vi "HFRR ADV v02.vi"() -> ()   [LabVIEW 2025] (continued)
            n899 = local write "Temperature Selection"(T15."Default" ("Temperature Selection")) -> ()
            n900 = local write "Calibration Selection"(T10."Default" ("Calibration Selection")) -> ()
            n901 = local write "Friction Force Tab"(T13."Page 1" ("Friction Force Tab")) -> ()
            n902 = local write "Main Calibration Tab"(T9."Main" ("Main Calibration Tab")) -> ()
            n903 = property on="Tab Control 6" class="TabCtl (strict)"("Visible"=FALSE) -> ()  [unwired: 2 in, 2 out]
            n904 = property on="Friction Force Calibration Result Tab" class="TabCtl (strict)"("Visible"=FALSE) -> ()  [unwired: 2 in, 2 out]
          }
        }
      }
      event "Accept & Save FF": Value Change {
        n905 = event-data() -> ()  [unwired: 1 in, 6 out]
        n906 = stacked-sequence {
          frame #0 {
            n907 = Wait (ms)(milliseconds to wait=u32 1000) -> ()  [unwired: 1 out]
          }
          frame #1 {
            n908 = local write "Due Write"("VC;0") -> ()
          }
          frame #2 {
            n909 = Wait (ms)(milliseconds to wait=u32 1000) -> ()  [unwired: 1 out]
          }
          frame #3 {
            n910 = local write "Due Write"("VC;0") -> ()
          }
          frame #4 {
            w931 = FALSE
            n911 = local write "FF BACK 2"(w931) -> ()
            n912 = local write "FF BACK 3"(w931) -> ()
            n913 = local write "FF BACK 4"(w931) -> ()
            n914 = local write "FF BACK 5"(w931) -> ()
            n915 = local write "FF BACK 6"(w931) -> ()
            n916 = local write "FF BACK"(w931) -> ()
          }
          frame #5 {
            n917 = Get Date/Time In Seconds() -> (seconds since 1Jan1904=w934:timestamp)
            n918 = Format Into String(format string="%<%m/%d/%Y %I:%M:%S %p>T", w934) -> (resulting string=w932:string)  [unwired: 2 in, 1 out]
            n919 = local write "FRICTION CALIBRATION"(w932) -> ()
          }
          frame #6 {
            n920 = local write "Temperature Selection"(T15."Default" ("Temperature Selection")) -> ()
            n921 = local write "Calibration Selection"(T10."Default" ("Calibration Selection")) -> ()
            n922 = local write "Friction Force Tab"(T13."Page 1" ("Friction Force Tab")) -> ()
            n923 = local write "Main Calibration Tab"(T9."Main" ("Main Calibration Tab")) -> ()
            n924 = local write "Save Button"(TRUE ("Save Button")) -> ()
            n925 = property on="Tab Control 6" class="TabCtl (strict)"("Visible"=FALSE) -> ()  [unwired: 2 in, 2 out]
            n926 = property on="Friction Force Calibration Result Tab" class="TabCtl (strict)"("Visible"=FALSE) -> ()  [unwired: 2 in, 2 out]
          }
        }
      }
      event "FF CONTINUE": Value Change {
        n927 = event-data() -> ()  [unwired: 1 in, 6 out]
        n928 = local write "FF CONTINUE"(FALSE ("FF CONTINUE")) -> ()
        n929 = local write "Friction Force Tab"(T13."Page 2" ("Friction Force Tab")) -> ()
      }
      event "FF CONTINUE 2": Value Change {
        n930 = event-data() -> ()  [unwired: 1 in, 6 out]
        n931 = local write "FF CONTINUE 2"(FALSE ("FF CONTINUE")) -> ()
        n932 = local write "Friction Force Tab"(T13."Page 3" ("Friction Force Tab")) -> ()
      }
      event "FF CONTINUE 3": Value Change {
        n933 = event-data() -> ()  [unwired: 1 in, 6 out]
        n934 = local write "FF CONTINUE 3"(FALSE ("FF CONTINUE")) -> ()
        n935 = local write "Friction Force Tab"(T13."Page 4" ("Friction Force Tab")) -> ()
      }
      event "FF CONTINUE 4": Value Change {
        n936 = event-data() -> ()  [unwired: 1 in, 6 out]
        n937 = local write "FF CONTINUE 4"(FALSE ("FF CONTINUE")) -> ()
        n938 = local write "Friction Force Tab"(T13."Page 5" ("Friction Force Tab")) -> ()
        n939 = property on="Friction Force Calibration Result Tab" class="TabCtl (strict)"("Visible"=FALSE) -> ()  [unwired: 2 in, 2 out]
      }
      event "FF CONTINUE 5": Value Change {
        n940 = event-data() -> ()  [unwired: 1 in, 6 out]
        n941 = local write "FF CONTINUE 5"(FALSE ("FF CONTINUE")) -> ()
        n942 = local write "Friction Force Tab"(T13."Page 6" ("Friction Force Tab")) -> ()
        n943 = property on="Friction Force Calibration Result Tab" class="TabCtl (strict)"("Visible"=FALSE) -> ()  [unwired: 2 in, 2 out]
        n944 = property on="Tab Control 6" class="TabCtl (strict)"("Visible"=FALSE) -> ()  [unwired: 2 in, 2 out]
      }
      event "Stroke Report Button": Value Change {
        n945 = event-data() -> ()  [unwired: 1 in, 6 out]
        n946 = local read "Point 5 - 1.0 mm"() -> (w956:bool)
        n947 = case shown="False" w956 {
          tunnel: [0.8 1.0] -> w955
          frame False {
          }
          frame True {
          }
        }
        n948 = local read "Machine Serial Number"() -> (w959:string)
        n949 = local read "USERNAME"() -> (w957:string)
        n950 = local write "Stroke Report Button"(FALSE ("Stroke Report Button")) -> ()
        n951 = call "Stroke Calibration Report.vi"("measured_value"=w955, "operator_name"=w957, "Instrument_serial Number"=w959) -> ()  [unwired: 7 in, 2 out]
      }
      event "Sample Report Button": Value Change {
        n952 = event-data() -> ()  [unwired: 1 in, 6 out]
        n953 = local read "Machine Serial Number"() -> (w965:string)
        n954 = local read "Sample 0deg temp"() -> (w962:dbl)
        n955 = local read "Sample 60deg temp"() -> (w963:dbl)
        n956 = local read "USERNAME"() -> (w964:string)
        n957 = call "Temperature Calibration Report.vi"("measured_60"=w963, "measured_zero"=w962, "operator_name"=w964, "Instrument_serial Number"=w965) -> ()  [unwired: 6 in, 2 out]
        n958 = local write "Sample Report Button"(FALSE ("Sample Report Button")) -> ()
      }
      event "Report Button FF": Value Change {
        n959 = event-data() -> ()  [unwired: 1 in, 6 out]
        n960 = local read "FF PASS"() -> (w970:bool)
        n961 = local read "Machine Serial Number"() -> (w973:string)
        n962 = Select(t="PASS", s=w970, f="FAIL") -> (s? t:f=w967:string)
        n963 = local read "USERNAME"() -> (w972:string)
        n964 = call "FF Calibration Report.vi"("pass_or_fail"=w967, "operator_name"=w972, "Instrument_serial Number"=w973) -> ()  [unwired: 7 in, 2 out]
        n965 = local write "Report Button FF"(FALSE ("Sample Report Button")) -> ()
      }
      event "Air Temperature Report Button": Value Change {
        n966 = event-data() -> ()  [unwired: 1 in, 6 out]
        n967 = local read "Machine Serial Number"() -> (w978:string)
        n968 = local read "Air 0deg temp"() -> (w975:dbl)
        n969 = local read "Air 60deg temp"() -> (w976:dbl)
        n970 = local read "USERNAME"() -> (w977:string)
        n971 = call "Air Temperature Calibration Report.vi"("measured_60"=w976, "measured_zero"=w975, "operator_name"=w977, "Instrument_serial Number"=w978) -> ()  [unwired: 6 in, 2 out]
        n972 = local write "Air Temperature Report Button"(FALSE ("Sample Report Button")) -> ()
      }
      event "Quit": Value Change {
        n973 = event-data() -> ()  [unwired: 1 in, 6 out]
      }
    }
    n974 = Wait (ms)(milliseconds to wait=u32 100) -> ()  [unwired: 1 out]
  }
  n975 = while {
    shift-right: [w981] -> _
    shift-left: "Enum - Selector" -> [w982]
    stop <- w983 stop-if-true
    # "Auto Start Logic Loop"
    n976 = case shown="\"close\"" w982 {
      tunnel: [w986 w992 w1020 w1055 w1085 Auto_Start_enum."Exit" ("Enum - Selector") Auto_Start_enum."Init" ("Enum - Selector")] -> w981
      frame "Init", Default {
        n977 = local read "Auto Start Test"() -> (w985:bool)
        n978 = Select(t=Auto_Start_enum."Humidity & Temperature On" ("Enum - Selector"), s=w985, f=Auto_Start_enum."Init") -> (s? t:f=w986:T17)
      }
      frame "Humidity & Temperature On" {
        n979 = stacked-sequence {
          tunnel: [_ _ _ _ _ _ Auto_Start_enum."Reach point" ("Enum - Selector")] -> w989
          frame #0 {
            w994 = T19."Disabled and Grayed Out" ("Disabled")
            w995 = TRUE ("Heater Button")
            n980 = property on="Humidity" class="Bool (strict)"("DisabledEnum"=w994) -> ()  [unwired: 2 in, 2 out]
            n981 = property on="Heater Button" class="Bool (strict)"("DisabledEnum"=w994) -> ()  [unwired: 2 in, 2 out]
            n982 = local write "Heater Button"(w995) -> ()
            n983 = local write "Humidity"(w995) -> ()
            n984 = property on="Heater Button" class="Bool (strict)"("Val(Sgnl)"=TRUE ("Value (Signaling)")) -> ()  [unwired: 2 in, 2 out]
          }
          frame #1 {
            n985 = Wait (ms)(milliseconds to wait=u32 3000) -> ()  [unwired: 1 out]
          }
          frame #2 {
            n986 = local read "Set Temp"() -> (w1001:dbl)
            n987 = Number To Fractional String(number=w1001, precision (6)=i16 2) -> (F-format string=w998:string)  [unwired: 2 in]
            n988 = Concatenate Strings("ST;" ("Command"), w998) -> (w999:string)
            n989 = local write "Due Write"(w999) -> ()
          }
          frame #3 {
            n990 = Wait (ms)(milliseconds to wait=u32 1500) -> ()  [unwired: 1 out]
          }
          frame #4 {
            (unwired) i16 2 ("precision (6)")
            n991 = local read "WriteHumidity"() -> (w1003:string[])
            n992 = local read "Set Rh"() -> (w1006:dbl)
            n993 = Number To Fractional String(number=w1006) -> (F-format string=w1007:string)  [unwired: 3 in]
            n994 = Concatenate Strings("M;" ("new element/subarray"), w1007) -> (w1008:string)
            n995 = Insert Into Array(array=w1003, new element=w1008) -> (w1004:string[])  [unwired: 1 in]
            n996 = local write "WriteHumidity"(w1004) -> ()
            n997 = local write "Due Write"("HE;1" ("Command")) -> ()
          }
          frame #5 {
            n998 = Wait (ms)(milliseconds to wait=u32 1500) -> ()  [unwired: 1 out]
          }
          frame #6 {
            w1011 = TRUE ("Reach point temp")
            n999 = local write "Reach point Humidity"(w1011) -> ()
            n1000 = local write "Reach point temp"(w1011) -> ()
          }
        }
        n1001 = local read "Auto Start Test"() -> (w991:bool)
        n1002 = Not(x=w991) -> (.not. x?=w990:bool)
        n1003 = Select(t=Auto_Start_enum."close", s=w990, f=w989) -> (s? t:f=w992:T17)
      }
      frame "Reach point" {
        w1021 = TRUE ("PAUSE")
        w1029 = 1.0 ("y")
        w1032 = 1.0 ("y")
        n1004 = local read "Set Temp"() -> (w1014:dbl)
        n1005 = local read "Set Humidity:"() -> (w1028:dbl)
        n1006 = local read "Humidity ( %RH )"() -> (w1033:dbl)
        n1007 = Add(x=w1014, y=w1032) -> (x+y=w1031:dbl)
        n1008 = Subtract(x=w1014, y=w1032) -> (x-y=w1030:dbl)
        n1009 = Add(x=w1028, y=w1029) -> (x+y=w1027:dbl)
        n1010 = Subtract(x=w1028, y=w1029) -> (x-y=w1026:dbl)
        n1011 = local read "TEMP"() -> (w1034:dbl)
        n1012 = In Range and Coerce(upper limit=w1027, x=w1033, lower limit=w1026) -> (In Range?=w1015:bool)  [unwired: 1 out]
        n1013 = In Range and Coerce(upper limit=w1031, x=w1034, lower limit=w1030) -> (In Range?=w1016:bool)  [unwired: 1 out]
        n1014 = disable-structure shown="Enabled" {
          disable-tunnel: w1015 -> [w1035 _]
          disable-tunnel: [w1035 TRUE] -> w1013
          frame Disabled {
            n1015 = case shown="True" w1035 {
              frame False {
              }
              frame True {
                n1016 = case shown="True" "Reach point Humidity" {
                  selector: "Reach point Humidity" -> [_ w1041]
                  frame False {
                  }
                  frame True {
                    n1017 = local read "EVENT LOG"() -> (w1038:string)
                    n1018 = Not(x=w1041) -> (.not. x?=w1040:bool)
                    n1019 = local write "Reach point Humidity"(w1040) -> ()
                    n1020 = call "Event Log.vi"("Content"="Target Humidity reached", "EVENT LOG"=w1038) -> ("EVENT LOG"=w1039:string)  [unwired: 8 in, 1 out]
                    n1021 = local write "EVENT LOG"(w1039) -> ()
                  }
                }
              }
            }
          }
          frame Enabled {
          }
        }
        n1022 = case shown="True" w1016 {
          frame False {
          }
          frame True {
            n1023 = case shown="True" "Reach point temp" {
              selector: "Reach point temp" -> [_ w1048]
              frame False {
              }
              frame True {
                n1024 = local read "EVENT LOG"() -> (w1045:string)
                n1025 = Not(x=w1048) -> (.not. x?=w1047:bool)
                n1026 = local write "Reach point temp"(w1047) -> ()
                n1027 = call "Event Log.vi"("Content"="Target Temperature reached", "EVENT LOG"=w1045) -> ("EVENT LOG"=w1046:string)  [unwired: 8 in, 1 out]
                n1028 = local write "EVENT LOG"(w1046) -> ()
              }
            }
          }
        }
        n1029 = local read "Auto Start Test"() -> (w1019:bool)
        n1030 = And(x=w1016, y=w1013) -> (x .and. y?=w1025:bool)
        n1031 = Select(t=Auto_Start_enum."Maintain Stage" ("Enum - Selector"), s=w1025, f=Auto_Start_enum."Reach point" ("Enum - Selector")) -> (s? t:f=w1022:T17)
        n1032 = Not(x=w1019) -> (.not. x?=w1018:bool)
        n1033 = Select(t=Auto_Start_enum."close", s=w1018, f=w1022) -> (s? t:f=w1020:T17)
        n1034 = call "ELAPSED TIMER VI.vi"("RESET"=w1021, "PAUSE"=w1021) -> ()  [unwired: 7 in, 3 out]
      }
      frame "Maintain Stage" {
        w1063 = 2.0 ("y")
        w1062 = 1.0 ("y")
        # "Humidity and temperature set point has stabilized."
        # "Humidity and  temperatures Set Point  have been reached"
        n1035 = local read "Set Temp"() -> (w1050:dbl)
        n1036 = local read "Set Humidity:"() -> (w1066:dbl)
        n1037 = local read "Humidity ( %RH )"() -> (w1069:dbl)
        n1038 = Add(x=w1050, y=w1062) -> (x+y=w1068:dbl)
        n1039 = Subtract(x=w1050, y=w1062) -> (x-y=w1067:dbl)
        n1040 = local read "TEMP"() -> (w1070:dbl)
        n1041 = Add(x=w1066, y=w1063) -> (x+y=w1065:dbl)
        n1042 = Subtract(x=w1066, y=w1063) -> (x-y=w1064:dbl)
        n1043 = In Range and Coerce(upper limit=w1068, x=w1070, lower limit=w1067) -> (In Range?=w1061:bool)  [unwired: 1 out]
        n1044 = In Range and Coerce(upper limit=w1065, x=w1069, lower limit=w1064) -> ()  [unwired: 2 out]
        n1045 = And(x=w1061, y=TRUE) -> (x .and. y?=w1060:bool)
        n1046 = Not(x=w1060) -> (.not. x?=w1059:bool)
        n1047 = call "ELAPSED TIMER VI.vi"("TARGET"=60.0, "RESET"=w1059, "PAUSE"=FALSE) -> ("ELAPSED INDICATION"=w1056:bool)  [unwired: 6 in, 2 out]
        n1048 = case shown="True" w1056 {
          tunnel: w1056 -> [_ w1073]
          tunnel: [Auto_Start_enum."Maintain Stage" ("Enum - Selector") w1072] -> w1054
          frame False {
          }
          frame True {
            n1049 = stacked-sequence {
              tunnel: w1073 -> [_ _ _ _ _]
              tunnel: [_ _ _ _ Auto_Start_enum."Start Stage" ("Enum - Selector")] -> w1072
              frame #0 {
                n1050 = local read "EVENT LOG"() -> (w1075:string)
                n1051 = call "Event Log.vi"("Content"="Temperature set point has stabilized.", "EVENT LOG"=w1075) -> ("EVENT LOG"=w1076:string)  [unwired: 8 in, 1 out]
                n1052 = local write "EVENT LOG"(w1076) -> ()
              }
              frame #1 {
                n1053 = Wait (ms)(milliseconds to wait=u32 100) -> ()  [unwired: 1 out]
              }
              frame #2 {
                n1054 = local read "EVENT LOG"() -> (w1080:string)
                n1055 = call "Event Log.vi"("Content"="Auto Test Started", "EVENT LOG"=w1080) -> ("EVENT LOG"=w1081:string)  [unwired: 8 in, 1 out]
                n1056 = local write "EVENT LOG"(w1081) -> ()
                n1057 = local write "FRICVALZ 4"(TRUE ("FRICVALZ 4")) -> ()
              }
              frame #3 {
                w1082 = TRUE ("RUN")
                n1058 = local write "RUN"(w1082) -> ()
                n1059 = property on="Auto Start Temp" class="Bool (strict)"("Val(Sgnl)"=w1082) -> ()  [unwired: 2 in, 2 out]
                "Auto Start Temp" <- w1082
              }
              frame #4 {
              }
            }
          }
        }
        n1060 = local read "Auto Start Test"() -> (w1053:bool)
        n1061 = Not(x=w1053) -> (.not. x?=w1052:bool)
        n1062 = Select(t=Auto_Start_enum."close", s=w1052, f=w1054) -> (s? t:f=w1055:T17)
      }
      frame "Start Stage" {
        w1084 = TRUE ("PAUSE")
        n1063 = local read "Auto Start Test"() -> (w1089:bool)
        n1064 = Not(x=w1089) -> (.not. x?=w1088:bool)
        n1065 = Select(t=Auto_Start_enum."close" ("Enum - Selector"), s=w1088, f=Auto_Start_enum."Start Stage" ("Enum - Selector")) -> (s? t:f=w1085:T17)
        n1066 = call "ELAPSED TIMER VI.vi"("RESET"=w1084, "PAUSE"=w1084) -> ()  [unwired: 7 in, 3 out]
      }
      frame "close" {
        w1092 = FALSE ("Heater Button")
        n1067 = local write "RUN"(w1092) -> ()
        n1068 = local write "Heater Button"(w1092) -> ()
        n1069 = local write "Humidity"(w1092) -> ()
        n1070 = local write "Auto Start Test"(w1092) -> ()
        n1071 = property on="Heater Button" class="Bool (strict)"("Val(Sgnl)"=FALSE ("Value (Signaling)")) -> ()  [unwired: 2 in, 2 out]
        n1072 = local write "Humidity 2"(TRUE ("Humidity")) -> ()
      }
      frame "Exit" {
      }
    }
    n1073 = Wait (ms)(milliseconds to wait=u32 100) -> ()  [unwired: 1 out]
    n1074 = local read "Quit"() -> (w983:bool)
  }
  n1075 = property on="Service Password Log" class="Str"("Visible"=w26) -> ()  [unwired: 2 in, 2 out]
  n1076 = property on="Password 3" class="Clust (strict)"("Visible"=w26) -> ()  [unwired: 2 in, 2 out]
  n1077 = while {
    stop <- w1121 stop-if-true
    w1104 = errorcluster {"status"=FALSE, "code"=0, "source"=""} ("error in (no error) 3")
    # "this loop is for manual report generation"
    n1078 = local read "Confirm Measrurement"() -> (w1103:bool)
    n1079 = case shown="True" w1103 {
      selector: w1103 -> [_ w1211]
      tunnel: errorcluster {"status"=FALSE, "code"=0, "source"=""} ("error in (no error) 3") -> [_ w1212]
      tunnel: [_ w1210] -> _
      frame False {
      }
      frame True {
        n1080 = stacked-sequence {
          tunnel: w1212 -> [_ w1245 _]
          tunnel: w1211 -> [_ _ w1354]
          tunnel: [_ w1233 _] -> w1210
          frame #0 {
            n1081 = String To Path(string="C:\\LAB-IQ\\Image Calibrate v01.dcf") -> (path=w1215:path)
            n1082 = Open/Create/Replace File ("Open File")(file path (use dialog)=w1215) -> (refnum out=w1216:refnum<file>)  [unwired: 5 in, 2 out]
            n1083 = for {
              N: 4 -> [_]
              tunnel: w1216 -> [w1222]
              i -> [w1218]
              n1084 = Read from Text File ("Read File")(file (use dialog)=w1222) -> (text=w1223:string)  [unwired: 3 in, 3 out]
              n1085 = String Subset(string=w1223, offset (0)=6, length (rest)=10 ("length (rest)")) -> (substring=w1219:string)
              n1086 = Fract/Exp String To Number(string=w1219) -> (number=w1217:dbl)  [unwired: 3 in, 1 out]
              n1087 = case shown="3" w1218 {
                tunnel: w1217 -> [w1224 w1225 _ w1226 _]
                frame 0 {
                  n1088 = local write "5x Gain"(w1224) -> ()
                }
                frame 1 {
                  n1089 = local write "10x Gain"(w1225) -> ()
                }
                frame 2 {
                }
                frame 3 {
                  n1090 = local write "100x gain"(w1226) -> ()
                }
                frame 4, Default {
                }
              }
            }
          }
          frame #1 {
            n1091 = local read "TEST STANDARD"() -> (w1228:T5)
            n1092 = case shown="\"ASTM D7688\"" w1228 {
              tunnel: ["ASTM D6079" "ISO 12156" "ASTM D7688"] -> w1227
              frame "ASTM D6079", Default {
              }
              frame "ISO 12156" {
              }
              frame "ASTM D7688" {
              }
            }
            n1093 = call "IMAGE ANALYSIS.vi"("Enum"=POST_ANALYSIS_ENUM."GET MEASUREMENTS", "error in"=w1245) -> ("error out"=w1252:errorcluster)  [unwired: 8 in, 1 out]
            n1094 = local read "Magnification :"() -> (w1238:string)
            n1095 = call "Stall Data Flow.vim"("value in"=w1252, "milliseconds to wait"=u32 1000) -> ("value out"=w1251:errorcluster)  [unwired: 1 out]
            n1096 = local read "Test File List :"() -> (w1249:string)
            n1097 = case shown="\"10x\"" w1238 {
              tunnel: [w1290 w1291] -> w1236
              frame "5x", Default {
                n1098 = local read "5x Gain"() -> (w1290:dbl)
              }
              frame "10x" {
                # "5x"
                n1099 = local read "10x Gain"() -> (w1291:dbl)
              }
            }
            n1100 = call "IMAGE ANALYSIS.vi"("Enum"=POST_ANALYSIS_ENUM."READ", "error in"=w1251) -> ("error out"=w1248:errorcluster, "data out"=w1239:string)  [unwired: 8 in]
            n1101 = Match Pattern(string=w1239, regular expression="\"type\": ") -> (after substring=w1243:string)  [unwired: 1 in, 3 out]
            n1102 = call "IMAGE PATH CREATION PY.vi"("error in (no error)"=w1248, "File Name :"=w1249) -> ("error out"=w1247:errorcluster, "File Path"=w1235:path, "File Path String:"=w1230:string)  [unwired: 7 in]
            n1103 = Match Pattern(string=w1243, regular expression=",") -> (before substring=w1229:string)  [unwired: 1 in, 3 out]
            n1104 = local read "Calibration Tab"() -> (w1232:enum32{"Measrument", "Calibrate"})
            n1105 = call "Stall Data Flow.vim"("value in"=w1247, "milliseconds to wait"=u32 250) -> ("value out"=w1231:errorcluster)  [unwired: 1 out]
            n1106 = Equal?(x=w1229, y="\"rectangle\"") -> (x = y?=w1240:bool)
            n1107 = case shown="False" w1240 {
              tunnel: w1239 -> [w1296 w1351]
              tunnel: w1236 -> [_ w1342]
              tunnel: cluster{"major":dbl, "minor":dbl, "average":dbl} {"major"=0.0, "minor"=0.0, "average"=0.0} -> [w1294 w1338]
              tunnel: [w1293 w1335] -> w1234
              tunnel: w1229 -> [w1295 _]
              tunnel: w1236 -> [w1292 _]
              frame False {
                n1108 = Equal?(x=w1295, y="\"line\"") -> (x = y?=w1297:bool)
                n1109 = case shown="True" w1297 {
                  tunnel: w1296 -> [_ w1312]
                  tunnel: w1294 -> [w1299 w1311]
                  tunnel: [w1299 w1309] -> w1293
                  tunnel: w1292 -> [_ w1308]
                  frame False {
                  }
                  frame True {
                    w1307 = 0.0 ("Major Axis")
                    n1110 = Match Pattern(string=w1312, regular expression="\"length_px\":") -> (after substring=w1310:string)  [unwired: 1 in, 3 out]
                    n1111 = property on="Major Axis" class="DigNum (strict)"("Caption.Text"="") -> ()  [unwired: 2 in, 2 out]
                    n1112 = property on="Minor Axis" class="DigNum (strict)"("Caption.Text"="") -> ()  [unwired: 2 in, 2 out]
                    n1113 = property on="Average" class="DigNum (strict)"("Caption.Text"="Line") -> ()  [unwired: 2 in, 2 out]
                    n1114 = Fract/Exp String To Number(string=w1310, default (0 dbl)=0.0 ("default (0 DBL)")) -> (number=w1306:dbl)  [unwired: 2 in, 1 out]
                    "Pixel Value" <- w1306
                    n1115 = Multiply(x=w1306, y=w1308) -> (x*y=w1319:dbl)
                    n1116 = Multiply(x=w1319, y=1000.0) -> (x*y=w1302:dbl)
                    n1117 = Divide(x=w1302, y=1000.0) -> (x/y=w1305:dbl)
                    n1118 = local write "Measurment (mm)"(w1305) -> ()
                    n1119 = Bundle By Name(cluster=w1311, "average"=w1302) -> (w1309:cluster{"major":dbl, "minor":dbl, "average":dbl})
                    n1120 = Number To Fractional String(number=w1302, precision (6)=i16 1) -> (F-format string=w1301:string)  [unwired: 2 in]
                    n1121 = local write "Minor Axis"(w1307) -> ()
                    n1122 = local write "Major Axis"(w1307) -> ()
                    n1123 = Fract/Exp String To Number(string=w1301) -> (number=w1300:dbl)  [unwired: 3 in, 1 out]
                    n1124 = local write "Average"(w1300) -> ()
                  }
                }
              }
              frame True {
                w1339 = 1000.0 ("y")
                w1345 = 0.0 ("default (0 DBL)")
                n1125 = Match Pattern(string=w1351, regular expression=" \"width_px\":") -> (after substring=w1349:string)  [unwired: 1 in, 3 out]
                n1126 = Match Pattern(string=w1349, regular expression="\"height_px\":") -> (before substring=w1347:string, after substring=w1346:string)  [unwired: 1 in, 2 out]
                n1127 = Fract/Exp String To Number(string=w1347, default (0 dbl)=w1345) -> (number=w1344:dbl)  [unwired: 2 in, 1 out]
                n1128 = Fract/Exp String To Number(string=w1346, default (0 dbl)=w1345) -> (number=w1343:dbl)  [unwired: 2 in, 1 out]
                n1129 = Multiply(x=w1344, y=w1342) -> (x*y=w1341:dbl)
                n1130 = Multiply(x=w1343, y=w1342) -> (x*y=w1340:dbl)
                n1131 = Multiply(x=w1341, y=w1339) -> (x*y=w1325:dbl)
                n1132 = Multiply(x=w1340, y=w1339) -> (x*y=w1323:dbl)
                n1133 = Add(x=w1325, y=w1323) -> (x+y=w1337:dbl)
                n1134 = property on="Major Axis" class="DigNum (strict)"("Caption.Text"="Major Axis") -> ()  [unwired: 2 in, 2 out]
                n1135 = property on="Minor Axis" class="DigNum (strict)"("Caption.Text"="Minor Axis") -> ()  [unwired: 2 in, 2 out]
                n1136 = property on="Average" class="DigNum (strict)"("Caption.Text"="Average") -> ()  [unwired: 2 in, 2 out]
                n1137 = Divide(x=w1337, y=2.0) -> (x/y=w1321:dbl)
                n1138 = Bundle By Name(cluster=w1338, "major"=w1325, "minor"=w1323, "average"=w1321) -> (w1335:cluster{"major":dbl, "minor":dbl, "average":dbl})
                n1139 = Number To Fractional String(number=w1323, precision (6)=i16 1) -> (F-format string=w1330:string)  [unwired: 2 in]
                n1140 = Number To Fractional String(number=w1321, precision (6)=i16 1) -> (F-format string=w1331:string)  [unwired: 2 in]
                n1141 = Number To Fractional String(number=w1325, precision (6)=i16 1) -> (F-format string=w1329:string)  [unwired: 2 in]
                n1142 = Fract/Exp String To Number(string=w1330) -> (number=w1322:dbl)  [unwired: 3 in, 1 out]
                n1143 = Fract/Exp String To Number(string=w1331) -> (number=w1320:dbl)  [unwired: 3 in, 1 out]
                n1144 = Fract/Exp String To Number(string=w1329) -> (number=w1324:dbl)  [unwired: 3 in, 1 out]
                n1145 = local write "Major Axis"(w1324) -> ()
                n1146 = local write "Average"(w1320) -> ()
                n1147 = local write "Minor Axis"(w1322) -> ()
              }
            }
            n1148 = case shown="\"Measrument\", Default" w1232 {
              tunnel: w1235 -> [w1263 _]
              tunnel: w1234 -> [w1262 _]
              tunnel: [w1259 w1289] -> w1233
              tunnel: w1231 -> [w1261 w1289]
              tunnel: w1230 -> [w1260 _]
              tunnel: w1227 -> [w1258 _]
              frame "Measrument", Default {
                n1149 = stacked-sequence {
                  tunnel: w1263 -> [w1282 _]
                  tunnel: w1262 -> [w1280 _]
                  tunnel: w1261 -> [w1278 _]
                  tunnel: w1260 -> [w1277 _]
                  tunnel: [w1272 _] -> w1259
                  tunnel: w1258 -> [w1265 _]
                  frame #0 {
                    n1150 = call "IMAGE ANALYSIS.vi"("Enum"=POST_ANALYSIS_ENUM."SAVE IMAGE", "error in"=w1278, "IMAGE FILE PATH"=w1277) -> ("error out"=w1276:errorcluster)  [unwired: 7 in, 1 out]
                    n1151 = call "Stall Data Flow.vim"("value in"=w1276, "milliseconds to wait"=u32 1000) -> ("value out"=w1267:errorcluster)  [unwired: 1 out]
                    n1152 = local read "Test File List :"() -> (w1284:string)
                    n1153 = call "IMAGE ANALYSIS.vi"("Enum"=POST_ANALYSIS_ENUM."MINIMIZE UI", "error in"=w1267) -> ("error out"=w1274:errorcluster)  [unwired: 8 in, 1 out]
                    n1154 = Bundle By Name(cluster=T26 {"File Name"="", "Test Method"="", "Operator"="", "Fuel Description"="", "Date and time"=""} ("Main Ref"), "Test Method"=w1265, "File Name"=w1284) -> (w1285:T26)
                    n1155 = call "Stall Data Flow.vim"("value in"=w1274, "milliseconds to wait"=u32 1500) -> ("value out"=w1269:errorcluster)  [unwired: 1 out]
                    n1156 = call "duf file read.vi"("error in (no error)"=w1269, "Main Ref"=w1285) -> ("error out"=w1283:errorcluster, "output cluster"=w1264:T27, "Main Ref 2"=w1281:T26)  [unwired: 7 in]
                    n1157 = call "DETECTION REPORT for manual.vi"("NEW PARAMETERS"=w1264, "error in (no error)"=w1283, "return value 3"=w1280, "Image File Path"=w1282, "Main Ref"=w1281) -> ("error out"=w1279:errorcluster)  [unwired: 6 in]
                    n1158 = call <vilib>:"Clear Errors.vi"("error in (no error)"=w1279) -> ("error out"=w1270:errorcluster)  [unwired: 5 in, 1 out]
                    n1159 = call "IMAGE ANALYSIS.vi"("Enum"=POST_ANALYSIS_ENUM."MINIMIZE UI", "error in"=w1270) -> ("error out"=w1272:errorcluster)  [unwired: 8 in, 1 out]
                  }
                  frame #1 {
                    n1160 = local write "Main Tab"(T4."HOME" ("Main Tab")) -> ()
                    n1161 = local write "Main Dashboard Buttons"(T1."Home" ("Main Dashboard Buttons")) -> ()
                  }
                }
              }
              frame "Calibrate" {
              }
            }
          }
          frame #2 {
            n1162 = Not(x=w1354) -> (.not. x?=w1353:bool)
            n1163 = local write "Confirm Measrurement"(w1353) -> ()
            n1164 = local read "Calibration Tab"() -> (w1352:enum32{"Measrument", "Calibrate"})
            n1165 = case shown="\"Measrument\", Default" w1352 {
              frame "Measrument", Default {
                (unwired) T21."HOME" ("Main Tab")
                n1166 = local write "Main Tab"(T4."HOME" ("Main Tab")) -> ()
              }
              frame "Calibrate" {
              }
            }
          }
        }
      }
    }
    n1167 = local read "Humidity"() -> (w1095:bool)
    n1168 = local read "Save Change"() -> (w1100:bool)
    n1169 = local read "Calibrate"() -> (w1101:bool)
    n1170 = local read "Auto Start Test"() -> (w1096:bool)
    n1171 = case shown="True" w1101 {
      selector: w1101 -> [_ w1208]
      frame False {
      }
      frame True {
        n1172 = Not(x=w1208) -> (.not. x?=w1207:bool)
        n1173 = local write "Calibrate"(w1207) -> ()
        n1174 = local write "Calibration Tab"(enum32{"Measrument", "Calibrate"}."Calibrate" ("Calibration Tab")) -> ()
      }
    }
    n1175 = case shown="True" w1100 {
      selector: w1100 -> [_ w1152]
      frame False {
      }
      frame True {
        n1176 = stacked-sequence {
          tunnel: w1152 -> [_ _ _ _ w1206]
          frame #0 {
            n1177 = call "IMAGE ANALYSIS.vi"("Enum"=POST_ANALYSIS_ENUM."HIDE UI") -> ()  [unwired: 9 in, 2 out]
          }
          frame #1 {
            n1178 = local read "100x gain"() -> (w1154:dbl)
            n1179 = local read "10x Gain"() -> (w1155:dbl)
            n1180 = local read "5x Gain"() -> (w1156:dbl)
            n1181 = Number To Fractional String(number=w1155, width (-)=i16 4, precision (6)=i16 7) -> (F-format string=w1177:string)  [unwired: 1 in]
            n1182 = Number To Fractional String(number=0.0, width (-)=i16 4, precision (6)=i16 7) -> (F-format string=w1172:string)  [unwired: 1 in]
            n1183 = Number To Fractional String(number=w1154, width (-)=i16 4, precision (6)=i16 7) -> (F-format string=w1160:string)  [unwired: 1 in]
            n1184 = Number To Fractional String(number=w1156, width (-)=i16 10 ("precision (6)"), precision (6)=i16 7) -> (F-format string=w1186:string)  [unwired: 1 in]
            n1185 = Concatenate Strings("[CH1]" ("string"), w1186, " - 5x Gain" ("string"), "\r") -> (w1176:string)
            n1186 = Concatenate Strings("[CH2]" ("string"), w1177, " - 10x Gain" ("string"), "\r") -> (w1175:string)
            n1187 = Concatenate Strings("[CH3]" ("string"), w1172, " - 20x Gain" ("string"), "\r") -> (w1166:string)
            n1188 = Concatenate Strings("[CH4]" ("string"), w1160, " - 100x Gain" ("string"), "\r") -> (w1159:string)
            n1189 = String To Path(string="C:\\LAB-IQ\\Image Calibrate v01.dcf") -> (path=w1189:path)
            n1190 = Concatenate Strings(w1176, w1175, w1166, w1159) -> (w1174:string)
            n1191 = call <vilib>:"Write Characters To File.vi"("append to file? (new file:F)"=FALSE, "character string"=w1174, "file path (dialog if empty)"=w1189) -> ()  [unwired: 2 in, 1 out]
          }
          frame #2 {
            n1192 = String To Path(string="C:\\LAB-IQ\\Image Calibrate v01.dcf") -> (path=w1192:path)
            n1193 = Open/Create/Replace File ("Open File")(file path (use dialog)=w1192) -> (refnum out=w1193:refnum<file>)  [unwired: 5 in, 2 out]
            n1194 = for {
              N: 4 -> [_]
              tunnel: w1193 -> [w1199]
              i -> [w1195]
              n1195 = Read from Text File ("Read File")(file (use dialog)=w1199) -> (text=w1200:string)  [unwired: 3 in, 3 out]
              n1196 = String Subset(string=w1200, offset (0)=6, length (rest)=10 ("length (rest)")) -> (substring=w1196:string)
              n1197 = Fract/Exp String To Number(string=w1196) -> (number=w1194:dbl)  [unwired: 3 in, 1 out]
              n1198 = case shown="3" w1195 {
                tunnel: w1194 -> [w1201 w1202 _ w1203 _]
                frame 0 {
                  n1199 = local write "5x Gain"(w1201) -> ()
                }
                frame 1 {
                  n1200 = local write "10x Gain"(w1202) -> ()
                }
                frame 2 {
                }
                frame 3 {
                  n1201 = local write "100x gain"(w1203) -> ()
                }
                frame 4, Default {
                }
              }
            }
          }
          frame #3 {
            n1202 = call "IMAGE ANALYSIS.vi"("Enum"=POST_ANALYSIS_ENUM."SHOW UI") -> ()  [unwired: 9 in, 2 out]
          }
          frame #4 {
            n1203 = Not(x=w1206) -> (.not. x?=w1205:bool)
            n1204 = local write "Save Change"(w1205) -> ()
          }
        }
      }
    }
    n1205 = case shown="False" w1096 {
      tunnel: w1095 -> [w1122 _]
      frame False {
        n1206 = case shown="True" w1122 {
          frame False {
          }
          frame True {
            n1207 = local read "Set Humidity:"() -> (w1126:dbl)
            n1208 = local read "Set Humidity:"() -> (w1129:dbl)
            n1209 = local read "Humidity ( %RH )"() -> (w1130:dbl)
            n1210 = Subtract(x=w1126, y=2.0) -> (x-y=w1124:dbl)
            n1211 = Add(x=w1129, y=2.0) -> (x+y=w1125:dbl)
            n1212 = In Range and Coerce(upper limit=w1125, x=w1130, lower limit=w1124) -> (In Range?=w1123:bool)  [unwired: 1 out]
            n1213 = case shown="True" w1123 {
              frame False {
              }
              frame True {
                n1214 = case shown="True" "Manual Humididty Reached" {
                  selector: "Manual Humididty Reached" -> [_ w1133]
                  frame False {
                  }
                  frame True {
                    n1215 = Not(x=w1133) -> (.not. x?=w1132:bool)
                    n1216 = local write "Manual Humididty Reached"(w1132) -> ()
                    n1217 = local read "EVENT LOG"() -> (w1135:string)
                    n1218 = call "Event Log.vi"("Content"="Target Humidity reached", "EVENT LOG"=w1135) -> ("EVENT LOG"=w1134:string)  [unwired: 8 in, 1 out]
                    n1219 = local write "EVENT LOG"(w1134) -> ()
                  }
                }
              }
            }
          }
        }
      }
      frame True {
        n1220 = local write "Manual Humididty Reached"(TRUE ("Manual Humididty Reached")) -> ()
      }
    }
    n1221 = local read "Cap Live Image"() -> (w1116:bool)
    n1222 = local read "SCAR MEASURMENT"() -> (w1119:enum32{"Auto Scar", "Manual Scar"})
    n1223 = Equal?(x=w1119, y=enum32{"Auto Scar", "Manual Scar"}."Manual Scar" ("SCAR MEASURMENT")) -> (x = y?=w1117:bool)
    n1224 = And(x=w1117, y=w1116) -> (x .and. y?=w1115:bool)
    n1225 = Wait (ms)(milliseconds to wait=u32 250) -> ()  [unwired: 1 out]
    n1226 = case shown="True" w1115 {
      selector: w1115 -> [_ w1440]
      frame False {
      }
      frame True {
        n1227 = stacked-sequence {
          tunnel: [_ _ _ w1459 _] -> _
          tunnel: w1440 -> [_ _ _ _ w1466]
          frame #0 {
            w1441 = 0.0
            n1228 = local write "Major Axis"(w1441) -> ()
            n1229 = local write "Minor Axis"(w1441) -> ()
            n1230 = local write "Average"(w1441) -> ()
          }
          frame #1 {
            n1231 = call "CAMERA LIVE FEED FGV.vi"("Enum - Menu"=CAMERA_LIVE_FEED_ENUM."CAMERA MINIMIZE") -> ()  [unwired: 9 in, 2 out]
          }
          frame #2 {
            n1232 = local read "Magnification len live scar"() -> (w1445:string)
            n1233 = case shown="\"10x\", Default" w1445 {
              tunnel: ["_10x" "_5x"] -> w1444
              frame "10x", Default {
              }
              frame "5x" {
              }
            }
            n1234 = local read "FILE 3"() -> (w1451:string)
            n1235 = call <vilib>:"Trim Whitespace.vi"("string"="C:\\LAB-IQ\\images\\") -> ("trimmed string"=w1453:string)  [unwired: 1 in]
            n1236 = String To Path(string=w1453) -> (path=w1452:path)
            n1237 = Concatenate Strings(w1451, w1444, ".png" ("string")) -> (w1450:string)
            n1238 = Build Path(base path=w1452, name or relative path=w1450) -> (appended path=w1449:path)
            n1239 = Path To String(path=w1449) -> (string=w1448:string)
            n1240 = call "CAMERA LIVE FEED FGV.vi"("Enum - Menu"=CAMERA_LIVE_FEED_ENUM."CAMERA SAVE", "Image Path"=w1448) -> ("error out"=w1446:errorcluster)  [unwired: 8 in, 1 out]
            n1241 = case shown="No Error" w1446 {
              frame No Error {
                n1242 = One Button Dialog(message="Image saved successfully") -> ()  [unwired: 1 in, 1 out]
              }
              frame Error {
              }
            }
          }
          frame #3 {
            n1243 = call "LIST FILE NAMES.vi"() -> ("error out"=w1461:errorcluster, "filenames"=w1458:string[])  [unwired: 10 in]
            n1244 = call "IMAGE ANALYSIS.vi"("Enum"=POST_ANALYSIS_ENUM."SHOW UI", "error in"=w1461) -> ("error out"=w1459:errorcluster)  [unwired: 8 in, 1 out]
            n1245 = property on="Test File List :" class="CmbBox"("Strings[]"=w1458) -> ()  [unwired: 2 in, 2 out]
          }
          frame #4 {
            (unwired) T25."Report" ("Main Dashboard Buttons")
            (unwired) T28."Report" ("Main Dashboard Buttons")
            n1246 = Not(x=w1466) -> (.not. x?=w1465:bool)
            n1247 = local write "Zoom Factore"(0.0 ("Zoom Factore")) -> ()
            n1248 = local write "Cap Live Image"(w1465) -> ()
            n1249 = local write "Main Tab"(T4."Adv Scar Report" ("Main Tab")) -> ()
            n1250 = property on="Cap Live Image" class="Bool (strict)"("BoolText.Text"="Capture Image" ("Boolean Text.Text")) -> ()  [unwired: 2 in, 2 out]
            n1251 = local write "Main Dashboard Buttons"(T1."Report" ("Main Dashboard Buttons")) -> ()
          }
        }
      }
    }
    n1252 = local read "change Gain"() -> (w1099:bool)
    n1253 = local read "Back Square"() -> (w1098:bool)
    n1254 = case shown="True" w1099 {
      selector: w1099 -> [_ w1143]
      frame False {
      }
      frame True {
        n1255 = stacked-sequence {
          tunnel: w1143 -> [_ w1151]
          frame #0 {
            n1256 = local read "Actual (µm)"() -> (w1147:dbl)
            n1257 = local read "Pixel Value"() -> (w1146:dbl)
            n1258 = local read "Magnification :"() -> (w1145:string)
            n1259 = Divide(x=w1147, y=w1146) -> (x/y=w1144:dbl)
            n1260 = case shown="\"10x\"" w1145 {
              tunnel: w1144 -> [w1148 w1149]
              frame "10x" {
                n1261 = local write "10x Gain"(w1148) -> ()
              }
              frame "5x", Default {
                n1262 = local write "5x Gain"(w1149) -> ()
              }
            }
          }
          frame #1 {
            n1263 = Not(x=w1151) -> (.not. x?=w1150:bool)
            n1264 = local write "change Gain"(w1150) -> ()
          }
        }
      }
    }
    n1265 = case shown="True" w1098 {
      selector: w1098 -> [_ w1141]
      frame False {
      }
      frame True {
        n1266 = Not(x=w1141) -> (.not. x?=w1140:bool)
        n1267 = local write "Back Square"(w1140) -> ()
        n1268 = local write "Calibration Tab"(enum32{"Measrument", "Calibrate"}."Measrument" ("Calibration Tab")) -> ()
      }
    }
    n1269 = local read "Rectangle Tool"() -> (w1110:bool)
    n1270 = local read "Clear ROI Tool"() -> (w1109:bool)
    n1271 = local read "Open Image"() -> (w1114:bool)
    n1272 = local read "line tool"() -> (w1111:bool)
    n1273 = local read "OUT"() -> (w1112:bool)
    n1274 = local read "In"() -> (w1113:bool)
    n1275 = case shown="True" w1114 {
      selector: w1114 -> [_ w1426]
      tunnel: [w1417 w1428] -> _
      tunnel: w1104 -> [w1417 w1427]
      frame False {
      }
      frame True {
        w1421 = "_5x" ("regular expression")
        n1276 = Not(x=w1426) -> (.not. x?=w1425:bool)
        n1277 = local write "Open Image"(w1425) -> ()
        n1278 = call "IMAGE ANALYSIS.vi"("Enum"=POST_ANALYSIS_ENUM."HIDE UI", "error in"=w1427) -> ("error out"=w1435:errorcluster)  [unwired: 8 in, 1 out]
        n1279 = call <vilib>:"Clear Errors.vi"("error in (no error)"=w1435) -> ("error out"=w1418:errorcluster)  [unwired: 5 in, 1 out]
        n1280 = call "File Dialog"("start path"=path "C:/LAB-IQ/images", "error in"=w1418) -> ("selected path"=w1420:path, "error out"=w1433:errorcluster)  [unwired: 10 in, 2 out]
        "Image path  2" <- w1420
        n1281 = call <vilib>:"Clear Errors.vi"("error in (no error)"=w1433) -> ("error out"=w1432:errorcluster)  [unwired: 5 in, 1 out]
        n1282 = call "IMAGE ANALYSIS.vi"("Enum"=POST_ANALYSIS_ENUM."OPEN FILE", "error in"=w1432, "File Path"=w1420) -> ("error out"=w1431:errorcluster)  [unwired: 7 in, 1 out]
        n1283 = call <vilib>:"Clear Errors.vi"("error in (no error)"=w1431) -> ("error out"=w1430:errorcluster)  [unwired: 5 in, 1 out]
        n1284 = call "IMAGE ANALYSIS.vi"("Enum"=POST_ANALYSIS_ENUM."SHOW UI", "error in"=w1430) -> ("error out"=w1428:errorcluster)  [unwired: 8 in, 1 out]
        n1285 = local write "Zoom Factore"(100.0 ("Zoom Factore")) -> ()
        n1286 = Strip Path(path=w1420) -> (name=w1423:string)  [unwired: 1 out]
        n1287 = Match Pattern(string=w1423, regular expression=w1421) -> (match substring=w1422:string)  [unwired: 1 in, 3 out]
        n1288 = Equal?(x=w1422, y=w1421) -> (x = y?=w1419:bool)
        n1289 = case shown="False" w1419 {
          frame False {
            n1290 = local write "Magnification :"("10x" ("Magnification :")) -> ()
          }
          frame True {
            n1291 = local write "Magnification :"("5x" ("Magnification :")) -> ()
          }
        }
      }
    }
    n1292 = case shown="True" w1112 {
      selector: w1112 -> [_ w1402]
      tunnel: w1104 -> [w1399 w1407]
      tunnel: [w1399 w1401] -> _
      frame False {
      }
      frame True {
        n1293 = Not(x=w1402) -> (.not. x?=w1400:bool)
        n1294 = local read "Zoom Factore"() -> (w1405:dbl)
        n1295 = local write "OUT"(w1400) -> ()
        n1296 = call "IMAGE ANALYSIS.vi"("Enum"=POST_ANALYSIS_ENUM."ZOOM OUT", "error in"=w1407) -> ("error out"=w1401:errorcluster)  [unwired: 8 in, 1 out]
        n1297 = Divide(x=w1405, y=1.2) -> (x/y=w1403:dbl)
        n1298 = local write "Zoom Factore"(w1403) -> ()
      }
    }
    n1299 = case shown="True" w1113 {
      selector: w1113 -> [_ w1411]
      tunnel: w1104 -> [w1408 w1416]
      tunnel: [w1408 w1409] -> _
      frame False {
      }
      frame True {
        n1300 = Not(x=w1411) -> (.not. x?=w1410:bool)
        n1301 = local read "Zoom Factore"() -> (w1414:dbl)
        n1302 = local write "In"(w1410) -> ()
        n1303 = call "IMAGE ANALYSIS.vi"("Enum"=POST_ANALYSIS_ENUM."ZOOM IN", "error in"=w1416) -> ("error out"=w1409:errorcluster)  [unwired: 8 in, 1 out]
        n1304 = Multiply(x=w1414, y=1.2) -> (x*y=w1412:dbl)
        n1305 = local write "Zoom Factore"(w1412) -> ()
      }
    }
    n1306 = case shown="True" w1109 {
      selector: w1109 -> [_ w1383]
      tunnel: w1104 -> [w1381 w1385]
      tunnel: [w1381 w1384] -> _
      frame False {
      }
      frame True {
        n1307 = Not(x=w1383) -> (.not. x?=w1382:bool)
        n1308 = local write "Clear ROI Tool"(w1382) -> ()
        n1309 = call "IMAGE ANALYSIS.vi"("Enum"=POST_ANALYSIS_ENUM."CLEAR ROI", "error in"=w1385) -> ("error out"=w1384:errorcluster)  [unwired: 8 in, 1 out]
      }
    }
    n1310 = case shown="True" w1111 {
      selector: w1111 -> [_ w1395]
      tunnel: w1104 -> [w1393 w1398]
      tunnel: [w1393 w1396] -> _
      frame False {
      }
      frame True {
        n1311 = Not(x=w1395) -> (.not. x?=w1394:bool)
        n1312 = local write "line tool"(w1394) -> ()
        n1313 = call "IMAGE ANALYSIS.vi"("Enum"=POST_ANALYSIS_ENUM."DRAW LINE", "error in"=w1398) -> ("error out"=w1396:errorcluster)  [unwired: 8 in, 1 out]
      }
    }
    n1314 = case shown="True" w1110 {
      selector: w1110 -> [_ w1389]
      tunnel: w1104 -> [w1387 w1391]
      tunnel: [w1387 w1390] -> _
      frame False {
      }
      frame True {
        n1315 = Not(x=w1389) -> (.not. x?=w1388:bool)
        n1316 = local write "Rectangle Tool"(w1388) -> ()
        n1317 = call "IMAGE ANALYSIS.vi"("Enum"=POST_ANALYSIS_ENUM."DRAW REC", "error in"=w1391) -> ("error out"=w1390:errorcluster)  [unwired: 8 in, 1 out]
      }
    }
    n1318 = local read "SCAR MEASURMENT"() -> (w1097:enum32{"Auto Scar", "Manual Scar"})
    n1319 = local read "Fit to Screen Tool"() -> (w1106:bool)
    n1320 = local read "Resize Tool"() -> (w1105:bool)
    n1321 = case shown="\"Manual Scar\", Default" w1097 {
      frame "Auto Scar" {
        n1322 = property on="Cap Live Image" class="Bool (strict)"("BoolText.Text"="Report" ("Boolean Text.Text")) -> ()  [unwired: 2 in, 2 out]
      }
      frame "Manual Scar", Default {
        n1323 = property on="Cap Live Image" class="Bool (strict)"("BoolText.Text"="Save Image" ("Boolean Text.Text")) -> ()  [unwired: 2 in, 2 out]
      }
    }
    n1324 = local read "ROI Color Tool"() -> (w1107:bool)
    n1325 = local read "Pan Tool"() -> (w1108:bool)
    n1326 = case shown="True" w1108 {
      selector: w1108 -> [_ w1377]
      tunnel: w1104 -> [w1375 w1379]
      tunnel: [w1375 w1378] -> _
      frame False {
      }
      frame True {
        n1327 = Not(x=w1377) -> (.not. x?=w1376:bool)
        n1328 = call "IMAGE ANALYSIS.vi"("Enum"=POST_ANALYSIS_ENUM."PAN", "error in"=w1379) -> ("error out"=w1378:errorcluster)  [unwired: 8 in, 1 out]
        n1329 = local write "Pan Tool"(w1376) -> ()
      }
    }
    n1330 = case shown="True" w1105 {
      selector: w1105 -> [_ w1361]
      tunnel: w1104 -> [w1356 w1358]
      tunnel: [w1356 w1357] -> _
      frame False {
      }
      frame True {
        n1331 = Not(x=w1361) -> (.not. x?=w1360:bool)
        n1332 = local write "Resize Tool"(w1360) -> ()
        n1333 = call "IMAGE ANALYSIS.vi"("Enum"=POST_ANALYSIS_ENUM."RESIZE MODE", "error in"=w1358) -> ("error out"=w1357:errorcluster)  [unwired: 8 in, 1 out]
      }
    }
    n1334 = case shown="True" w1106 {
      selector: w1106 -> [_ w1366]
      tunnel: [w1362 w1367] -> _
      tunnel: w1104 -> [w1362 w1365]
      frame False {
      }
      frame True {
        n1335 = Not(x=w1366) -> (.not. x?=w1364:bool)
        n1336 = local write "Zoom Factore"(100.0 ("Zoom Factore")) -> ()
        n1337 = local write "Fit to Screen Tool"(w1364) -> ()
        n1338 = call "IMAGE ANALYSIS.vi"("Enum"=POST_ANALYSIS_ENUM."FIT", "error in"=w1365) -> ("error out"=w1367:errorcluster)  [unwired: 8 in, 1 out]
      }
    }
    n1339 = case shown="True" w1107 {
      selector: w1107 -> [_ w1372]
      tunnel: [w1369 w1373] -> _
      tunnel: w1104 -> [w1369 w1370]
      frame False {
      }
      frame True {
        n1340 = Not(x=w1372) -> (.not. x?=w1371:bool)
        n1341 = local write "ROI Color Tool"(w1371) -> ()
        n1342 = call "IMAGE ANALYSIS.vi"("Enum"=POST_ANALYSIS_ENUM."SET ROI COLOR", "error in"=w1370) -> ("error out"=w1373:errorcluster)  [unwired: 8 in, 1 out]
      }
    }
    n1343 = local read "Quit"() -> (w1121:bool)
  }
  n1344 = while {
    stop <- w1468 stop-if-true
    n1345 = local read "Image Path"() -> (w1471:path)
    n1346 = local read "Print 3"() -> (w1474:bool)
    n1347 = Equal?(x=w1471, y=path "") -> (x = y?=w1470:bool)
    n1348 = Not(x=w1470) -> (.not. x?=w1469:bool)
    n1349 = property on="Print 3" class="Bool (strict)"("Visible"=w1469) -> ()  [unwired: 2 in, 2 out]
    n1350 = case shown="True" w1474 {
      frame False {
        n1351 = local write "Rd"(TRUE ("Boolean 7")) -> ()
      }
      frame True {
        n1352 = flat-sequence {
          tunnel: [w1514] -> w1482
          tunnel: [w1501] -> w1480
          tunnel: [w1511] -> w1476
          tunnel: w1482 -> [w1523]
          tunnel: [w1523] -> w1481
          tunnel: w1480 -> [w1522]
          tunnel: [w1522] -> w1479
          tunnel: [w1520] -> w1478
          tunnel: [w1519] -> w1477
          tunnel: w1476 -> [w1519]
          tunnel: w1481 -> [w1525]
          tunnel: w1479 -> [w1526]
          tunnel: w1478 -> [_]
          tunnel: w1477 -> [w1524]
          frame #0 {
            n1353 = case shown="True" "Rd" {
              frame False {
              }
              frame True {
                n1354 = while {
                  tunnel: "abcdefABCDEF" ("string 2") -> [w1493]
                  shift-right: [w1491] -> w1485
                  shift-left: "" -> [w1490]
                  i -> [w1500]
                  stop <- w1499 stop-if-true
                  n1355 = Random Number (0-1)() -> (number: 0 to 1=w1494:dbl)
                  n1356 = Multiply(x=w1494, y=62.0) -> (x*y=w1496:dbl)
                  n1357 = Decrement(x="Length 2") -> (x-1=w1489:i16)
                  n1358 = To Word Integer(number=w1496) -> (16bit integer=w1497:i16)
                  n1359 = String Subset(string=w1493, offset (0)=w1497, length (rest)=1 ("length (rest)")) -> (substring=w1492:string)
                  n1360 = Greater Or Equal?(x=w1500, y=w1489) -> (x >= y?=w1499:bool)
                  n1361 = Concatenate Strings(w1492, w1490) -> (w1491:string)
                }
                "String 10" <- w1485
                n1362 = local write "Rd"(FALSE ("Boolean 7")) -> ()
              }
            }
          }
          frame #1 {
            w1512 = "_resized.jpg" ("command line")
            (unwired) ".jpg -resize 320x240 " ("string")
            (unwired) "Choose an Image File" ("prompt")
            # "-resize 1798x425"
            n1363 = local read "Image Path"() -> (w1506:path)
            n1364 = Strip Path(path=w1506) -> (stripped path=w1501:path, name=w1502:string)
            n1365 = Match Pattern(string=w1502, regular expression=".jpg") -> (before substring=→"before substring 2":string, after substring=→"after substring":string)  [unwired: 1 in, 2 out]
            n1366 = Match Pattern(string=w1502, regular expression="\\") -> (before substring=w1508:string)  [unwired: 1 in, 3 out]
            n1367 = Match Pattern(string=w1508, regular expression=".jpg") -> (before substring=w1507:string)  [unwired: 1 in, 3 out]
            n1368 = Concatenate Strings("cmd /c convert " ("string"), w1507, ".jpg -resize 320x240  " ("command line"), w1507, w1512) -> (w1515:string)
            n1369 = call <vilib>:"System Exec.vi"("run minimized? (F)"=TRUE, "wait until completion? (T)"=TRUE, "working directory"=w1501, "command line"=w1515) -> ("error out"=w1514:errorcluster)  [unwired: 4 in, 3 out]
            "error out 2" <- w1514
            n1370 = Concatenate Strings(w1507, w1512) -> (w1511:string)
          }
          frame #2 {
            n1371 = Wait (ms)(milliseconds to wait=u32 2000 ("millisecond timer value")) -> (millisecond timer value=w1520:u32)
          }
          frame #3 {
            n1372 = case shown="No Error" w1525 {
              tunnel: w1526 -> [w1529 _]
              tunnel: w1524 -> [w1527 _]
              frame No Error {
                (unwired) ".jpg" ("string")
                n1373 = Path To String(path=w1529) -> (string=w1533:string)
                n1374 = Concatenate Strings(w1533, "\\" ("string"), w1527) -> (w1532:string)
                n1375 = String To Path(string=w1532) -> (path=w1531:path)
                n1376 = call <vilib>:"Read JPEG File.vi"("path to JPEG file"=w1531) -> ("image data"=w1535:T2)  [unwired: 8 in, 2 out]
                "image data" <- w1535
                n1377 = local write "Print 3"(FALSE ("Print 2")) -> ()
                n1378 = call <vilib>:"Draw Flattened Pixmap.vi"("image data"=w1535) -> ("new picture"=→"new picture":picture)  [unwired: 8 in]
              }
              frame Error {
              }
            }
          }
        }
      }
    }
    n1379 = Wait (ms)(milliseconds to wait=u32 20 ("millisecond timer value")) -> ()  [unwired: 1 out]
    n1380 = local read "Quit"() -> (w1468:bool)
  }
  n1381 = while {
    tunnel: w43 -> [_]
    tunnel: w29 -> [_]
    stop <- w1565 stop-if-true
    # "New Adv Logics"
    n1382 = local read "Main Tab"() -> (w1546:T4)
    n1383 = local read "Main Tab"() -> (w1563:T4)
    n1384 = local read "Sign In"() -> (w1562:bool)
    n1385 = case shown="\"Adv Scar\"" w1546 {
      frame "HOME", Default {
        n1386 = local read "LIVE FEED MIN TEMP"() -> (w1699:bool)
        n1387 = local write "LIVE FEED MAX TEMP"(TRUE ("LIVE FEED MAX TEMP")) -> ()
        n1388 = local read "CAMERA ROI MIN TEMP"() -> (w1697:bool)
        n1389 = case shown="True" w1699 {
          selector: w1699 -> [_ w1706]
          frame False {
          }
          frame True {
            n1390 = Not(x=w1706) -> (.not. x?=w1705:bool)
            n1391 = local write "LIVE FEED MIN TEMP"(w1705) -> ()
            n1392 = call "CAMERA LIVE FEED FGV.vi"("Enum - Menu"=CAMERA_LIVE_FEED_ENUM."CAMERA MINIMIZE") -> ()  [unwired: 9 in, 2 out]
          }
        }
        n1393 = case shown="True" w1697 {
          selector: w1697 -> [_ w1703]
          frame False {
          }
          frame True {
            n1394 = Not(x=w1703) -> (.not. x?=w1702:bool)
            n1395 = local write "CAMERA ROI MIN TEMP"(w1702) -> ()
            n1396 = call "IMAGE ANALYSIS.vi"("Enum"=POST_ANALYSIS_ENUM."MINIMIZE UI") -> ()  [unwired: 9 in, 2 out]
          }
        }
        n1397 = local write "CAMERA ROI MAX TEMP"(TRUE ("CAMERA ROI MAX TEMP")) -> ()
      }
      frame "Test Setup" {
        n1398 = local read "LIVE FEED MIN TEMP"() -> (w1709:bool)
        n1399 = local read "CAMERA ROI MIN TEMP"() -> (w1707:bool)
        n1400 = local write "LIVE FEED MAX TEMP"(TRUE ("LIVE FEED MAX TEMP")) -> ()
        n1401 = case shown="True" w1709 {
          selector: w1709 -> [_ w1716]
          frame False {
          }
          frame True {
            n1402 = Not(x=w1716) -> (.not. x?=w1715:bool)
            n1403 = local write "LIVE FEED MIN TEMP"(w1715) -> ()
            n1404 = call "CAMERA LIVE FEED FGV.vi"("Enum - Menu"=CAMERA_LIVE_FEED_ENUM."CAMERA MINIMIZE") -> ()  [unwired: 9 in, 2 out]
          }
        }
        n1405 = case shown="True" w1707 {
          selector: w1707 -> [_ w1713]
          frame False {
          }
          frame True {
            n1406 = Not(x=w1713) -> (.not. x?=w1712:bool)
            n1407 = local write "CAMERA ROI MIN TEMP"(w1712) -> ()
            n1408 = call "IMAGE ANALYSIS.vi"("Enum"=POST_ANALYSIS_ENUM."MINIMIZE UI") -> ()  [unwired: 9 in, 2 out]
          }
        }
        n1409 = local write "CAMERA ROI MAX TEMP"(TRUE ("CAMERA ROI MAX TEMP")) -> ()
      }
      frame "Acquire" {
        n1410 = local read "LIVE FEED MIN TEMP"() -> (w1719:bool)
        n1411 = local write "LIVE FEED MAX TEMP"(TRUE ("LIVE FEED MAX TEMP")) -> ()
        n1412 = local read "CAMERA ROI MIN TEMP"() -> (w1717:bool)
        n1413 = case shown="True" w1719 {
          selector: w1719 -> [_ w1726]
          frame False {
          }
          frame True {
            n1414 = Not(x=w1726) -> (.not. x?=w1725:bool)
            n1415 = local write "LIVE FEED MIN TEMP"(w1725) -> ()
            n1416 = call "CAMERA LIVE FEED FGV.vi"("Enum - Menu"=CAMERA_LIVE_FEED_ENUM."CAMERA MINIMIZE") -> ()  [unwired: 9 in, 2 out]
          }
        }
        n1417 = case shown="True" w1717 {
          selector: w1717 -> [_ w1723]
          frame False {
          }
          frame True {
            n1418 = Not(x=w1723) -> (.not. x?=w1722:bool)
            n1419 = local write "CAMERA ROI MIN TEMP"(w1722) -> ()
            n1420 = call "IMAGE ANALYSIS.vi"("Enum"=POST_ANALYSIS_ENUM."MINIMIZE UI") -> ()  [unwired: 9 in, 2 out]
          }
        }
        n1421 = local write "CAMERA ROI MAX TEMP"(TRUE ("CAMERA ROI MAX TEMP")) -> ()
      }
      frame "Adv Scar" {
        n1422 = local read "CAMERA ROI MIN TEMP"() -> (w1727:bool)
        n1423 = case shown="True" "LIVE FEED MAX TEMP" {
          selector: "LIVE FEED MAX TEMP" -> [_ w1748]
          frame False {
          }
          frame True {
            n1424 = Not(x=w1748) -> (.not. x?=w1747:bool)
            n1425 = local write "LIVE FEED MAX TEMP"(w1747) -> ()
            n1426 = call "CAMERA LIVE FEED FGV.vi"("Enum - Menu"=CAMERA_LIVE_FEED_ENUM."CAMERA RESTORE") -> ("error out"=w1738:errorcluster)  [unwired: 9 in, 1 out]
            n1427 = Type Cast(type=30, x=0) -> (*(type *) &x=w1742:i32)
            n1428 = Add(x=w1742, y=48) -> (x+y=w1743:i32)
            n1429 = call "CAMERA LIVE FEED FGV.vi"("Enum - Menu"=CAMERA_LIVE_FEED_ENUM."CAMERA MODE SET", "error in (no error)"=w1738, "CAMERA MODE"=w1743) -> ("error out"=w1735:errorcluster)  [unwired: 7 in, 1 out]
            n1430 = call "CAMERA LIVE FEED FGV.vi"("Enum - Menu"=CAMERA_LIVE_FEED_ENUM."CAMERA GRAY", "error in (no error)"=w1735) -> ("error out"=w1734:errorcluster)  [unwired: 8 in, 1 out]
            n1431 = call "LIST FILE NAMES.vi"("error in (no error)"=w1734) -> ("error out"=w1744:errorcluster, "filenames"=w1745:string[])  [unwired: 9 in]
            n1432 = property on="FILE 3" class="CmbBox"(error in=w1744, "Strings[]"=w1745) -> ()  [unwired: 1 in, 2 out]
          }
        }
        n1433 = case shown="True" w1727 {
          selector: w1727 -> [_ w1733]
          frame False {
          }
          frame True {
            n1434 = Not(x=w1733) -> (.not. x?=w1732:bool)
            n1435 = local write "CAMERA ROI MIN TEMP"(w1732) -> ()
            n1436 = call "IMAGE ANALYSIS.vi"("Enum"=POST_ANALYSIS_ENUM."MINIMIZE UI") -> ()  [unwired: 9 in, 2 out]
          }
        }
        n1437 = local write "CAMERA ROI MAX TEMP"(TRUE ("CAMERA ROI MAX TEMP")) -> ()
        "LIVE FEED MIN TEMP" <- TRUE ("LIVE FEED MIN TEMP")
      }
      frame "Adv Scar Report" {
        n1438 = local read "CAMERA ROI MAX TEMP"() -> (w1749:bool)
        n1439 = local read "LIVE FEED MIN TEMP"() -> (w1751:bool)
        n1440 = local write "LIVE FEED MAX TEMP"(TRUE ("LIVE FEED MAX TEMP")) -> ()
        n1441 = case shown="True" w1751 {
          selector: w1751 -> [_ w1760]
          frame False {
          }
          frame True {
            n1442 = Not(x=w1760) -> (.not. x?=w1759:bool)
            n1443 = local write "LIVE FEED MIN TEMP"(w1759) -> ()
            n1444 = call "CAMERA LIVE FEED FGV.vi"("Enum - Menu"=CAMERA_LIVE_FEED_ENUM."CAMERA MINIMIZE") -> ()  [unwired: 9 in, 2 out]
          }
        }
        n1445 = case shown="True" w1749 {
          selector: w1749 -> [_ w1757]
          frame False {
          }
          frame True {
            n1446 = Not(x=w1757) -> (.not. x?=w1755:bool)
            n1447 = local write "CAMERA ROI MAX TEMP"(w1755) -> ()
            n1448 = call "IMAGE ANALYSIS.vi"("Enum"=POST_ANALYSIS_ENUM."SHOW UI") -> ("error out"=w1754:errorcluster)  [unwired: 9 in, 1 out]
            n1449 = call "LIST FILE NAMES.vi"("error in (no error)"=w1754) -> ("filenames"=w1753:string[])  [unwired: 9 in, 1 out]
            n1450 = property on="Test File List :" class="CmbBox"("Strings[]"=w1753) -> ()  [unwired: 2 in, 2 out]
          }
        }
        n1451 = local write "CAMERA ROI MIN TEMP"(TRUE ("CAMERA ROI MIN TEMP")) -> ()
      }
      frame "Compare Files" {
        n1452 = local read "LIVE FEED MIN TEMP"() -> (w1763:bool)
        n1453 = local write "LIVE FEED MAX TEMP"(TRUE ("LIVE FEED MAX TEMP")) -> ()
        n1454 = local read "CAMERA ROI MIN TEMP"() -> (w1761:bool)
        n1455 = case shown="True" w1763 {
          selector: w1763 -> [_ w1770]
          frame False {
          }
          frame True {
            n1456 = Not(x=w1770) -> (.not. x?=w1769:bool)
            n1457 = local write "LIVE FEED MIN TEMP"(w1769) -> ()
            n1458 = call "CAMERA LIVE FEED FGV.vi"("Enum - Menu"=CAMERA_LIVE_FEED_ENUM."CAMERA MINIMIZE") -> ()  [unwired: 9 in, 2 out]
          }
        }
        n1459 = case shown="True" w1761 {
          selector: w1761 -> [_ w1767]
          frame False {
          }
          frame True {
            n1460 = Not(x=w1767) -> (.not. x?=w1766:bool)
            n1461 = local write "CAMERA ROI MIN TEMP"(w1766) -> ()
            n1462 = call "IMAGE ANALYSIS.vi"("Enum"=POST_ANALYSIS_ENUM."MINIMIZE UI") -> ()  [unwired: 9 in, 2 out]
          }
        }
        n1463 = local write "CAMERA ROI MAX TEMP"(TRUE ("CAMERA ROI MAX TEMP")) -> ()
      }
      frame "About" {
        n1464 = local read "LIVE FEED MIN TEMP"() -> (w1773:bool)
        n1465 = local write "LIVE FEED MAX TEMP"(TRUE ("LIVE FEED MAX TEMP")) -> ()
